vi "GetRoutes.vi"(8 "error in (no error)":errorcluster, 11 "reference in":refnum<class "SwitchBase.lvclass">) -> (0 "error out":errorcluster, 2 "Routes":T1[](array[typedef]), 3 "reference in":refnum<class "SwitchBase.lvclass">)   [LabVIEW 2022 SP3, in "SwitchBase.lvlib" / "SwitchBase.lvclass"]
uses:
  SwitchBase.lvclass
  Route.ctl
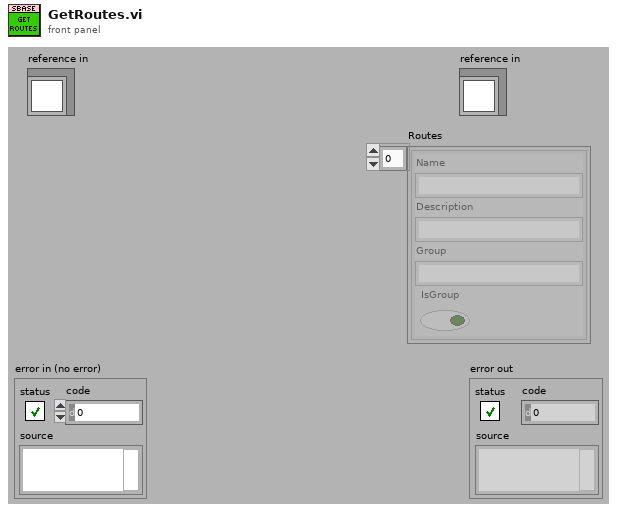
[diagram p1: front panel]
types:
  T1 = typedef "SwitchBase.lvlib/SwitchBase.lvclass/Route.ctl" = cluster{"Name":string, "Description":string, "Group":string, "IsGroup":bool}
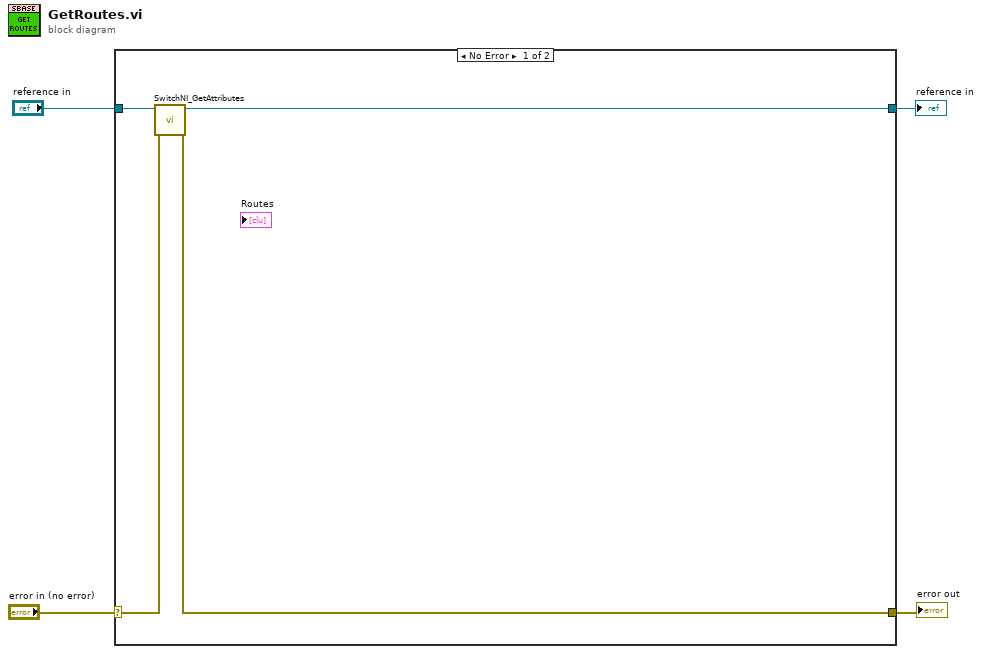
[diagram p0: block diagram]
diagram:
  n1 = case shown="No Error" "error in (no error)" {
    selector: "error in (no error)" -> [w8 w10]
    tunnel: [w7 w10] -> w3
    tunnel: [w5 w9] -> w1
    tunnel: "reference in" -> [w6 w9]
    frame No Error {
      n2 = call "SwitchNI_GetAttributes.vi"("error in (no error)"=w8, "reference in"=w6) -> ("error out"=w7:errorcluster, "reference out"=w5:refnum<class "SwitchBase.lvclass">)  [unwired: 6 in, 2 out]
    }
    frame Error {
    }
  }
  "error out" <- w3
  "reference in" <- w1
